vi "2D raster.vi"(11 "Scanning Parameters":T1={"x pixels"=16, "x voltage min"=-8.0, "x voltage max"=8.0, "y pixels"=16, "y voltage min"=-8.0, "y voltage max"=8.0, "x pts flyback"=16, "y pts flyback"=0, "Zoom"=1.0}) -> (1 "X and Y":waveform(dbl)[](graph)=[{"t0"=timestamp(0 s since 1904-01-01), "dt"=1.0, "Y"=array[512 elements]}, {"t0"=timestamp(0 s since 1904-01-01), "dt"=1.0, "Y"=array[512 elements]}], 2 "Y":waveform(dbl)(graph)={"t0"=timestamp(0 s since 1904-01-01), "dt"=1.0, "Y"=array[512 elements]}, 3 "X":waveform(dbl)(graph)={"t0"=timestamp(0 s since 1904-01-01), "dt"=1.0, "Y"=array[512 elements]})   [LabVIEW 2012]
panel:
  out "flyback":dbl[](graph)=[-8.0, -8.0, -8.0, -8.0, -8.0, -8.0, -10.0, -10.0, -10.0, -10.0, -10.0, -10.0, -10.0, -10.0, -10.0, -9.066666666666666]
  out "fast axis size":i32=512
  out "slow scan size":i32=512
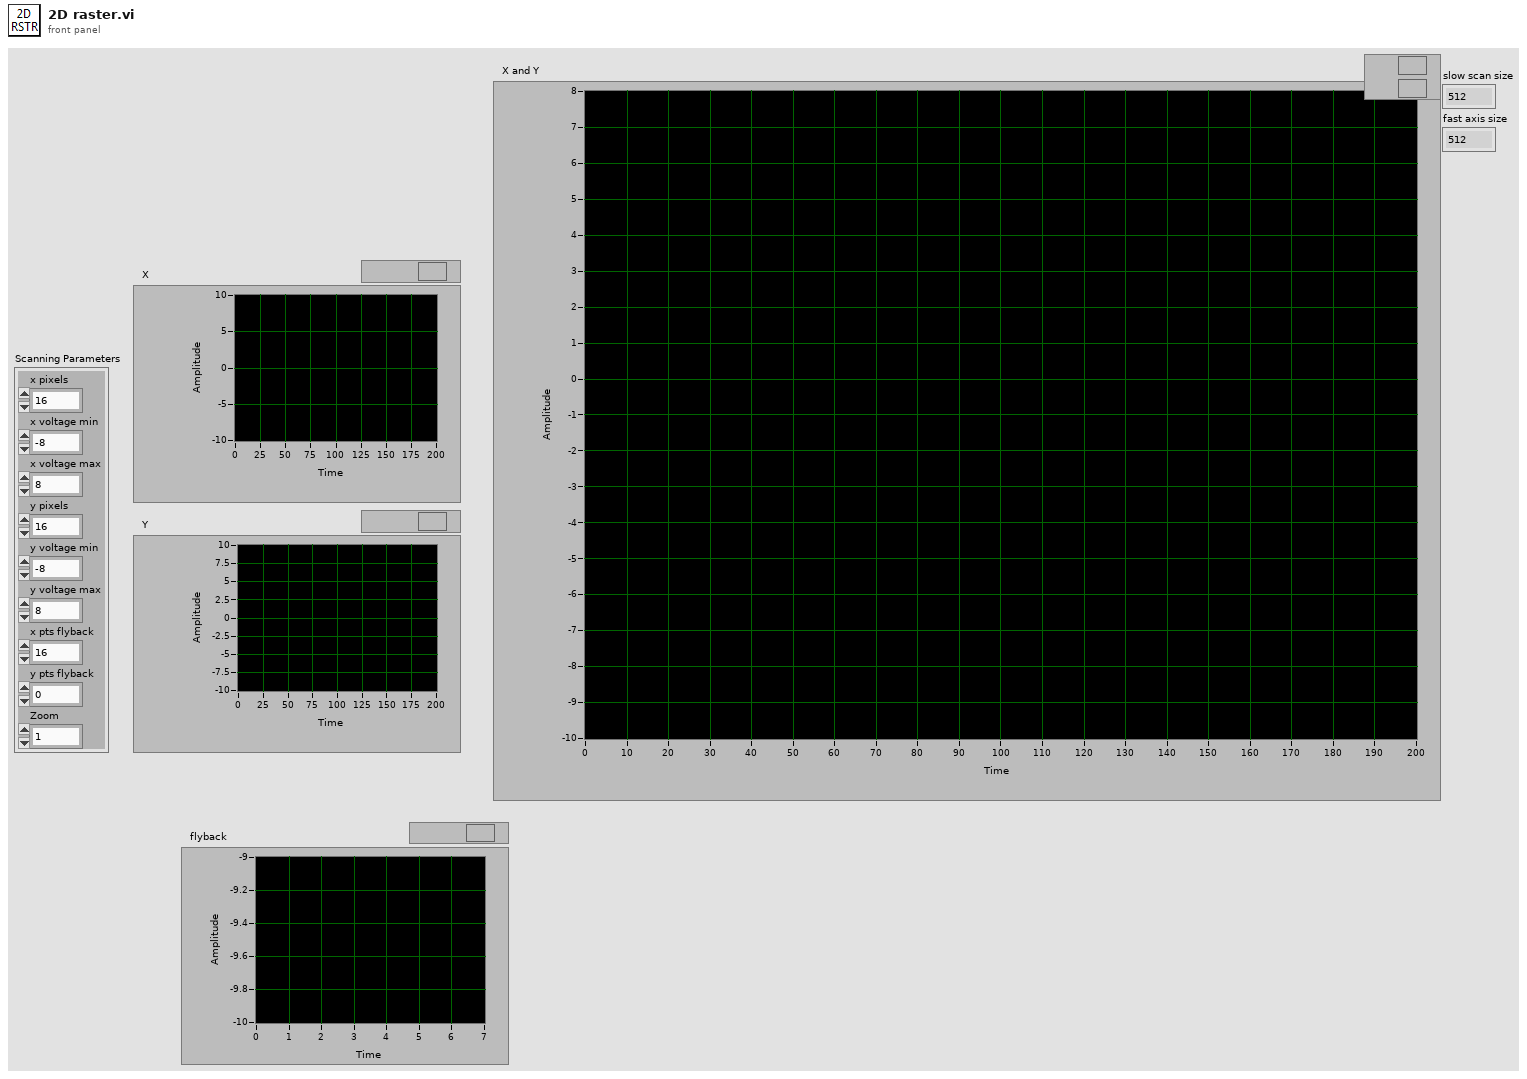
[diagram p1: front panel]
types:
  T1 = cluster{"x pixels":i32, "x voltage min":dbl, "x voltage max":dbl, "y pixels":i32, "y voltage min":dbl, "y voltage max":dbl, "x pts flyback":i32, "y pts flyback":i32, "Zoom":dbl}
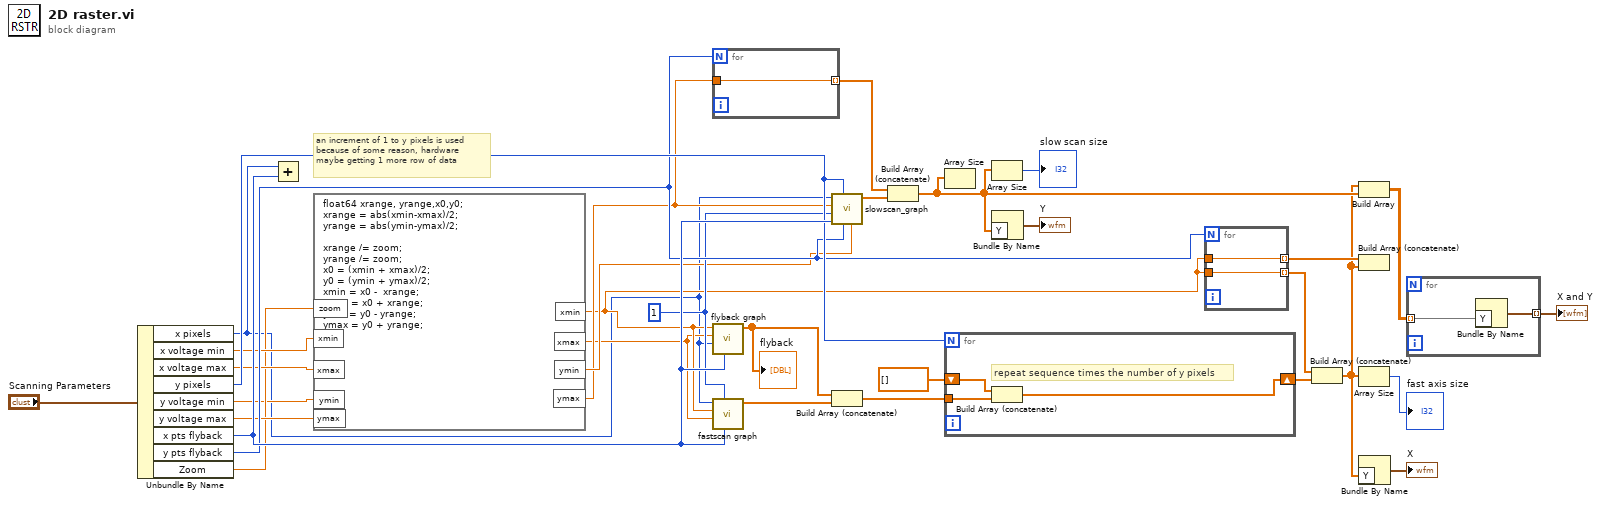
[diagram p0: block diagram]
diagram:
  w14 = 1 ("Samples to Average")
  # "an increment of 1 to y pixels is used\nbecause of some reason, hardware maybe getting 1 more row of data"
  n1 = Unbundle By Name("Scanning Parameters") -> ("x pixels"=w4:i32, "x voltage min"=w13:dbl, "x voltage max"=w12:dbl, "y pixels"=w26:i32, "y voltage min"=w9:dbl, "y voltage max"=w11:dbl, "x pts flyback"=w27:i32, "y pts flyback"=w25:i32, "Zoom"=w10:dbl)
  n2 = Add(x=w4, y=w27) -> ()  [unwired: 1 out]
  n3 = formula code="float64 xrange, yrange,x0,y0;\nxrange = abs(xmin-xmax)/2;\nyrange = abs(ymin-ymax)/2;\n\nxrange /= zoom;\nyrange /= zoom;\nx0 = (xmin + xmax)/2;\ny0 = (ymin + ymax)/2;\nxmin = x0 -  xrange;\nxmax = x0 + xrange;\nymin = y0 - yrange;\nymax = y0 + yrange;"("xmin"=w13, "xmax"=w12, "ymin"=w9, "ymax"=w11, "zoom"=w10) -> ("xmin"=w6:dbl, "xmax"=w5:dbl, "ymin"=w8:dbl, "ymax"=w7:dbl)
  n4 = for {
    N: w25 -> [_]
    tunnel: w7 -> [w33]
    tunnel: [w33] -> w24 mode=indexing
  }
  n5 = call "flyback graph.vi"("x pts flyback"=w27, "x pixels"=w4, "x max"=w5, "x min"=w6) -> ("Array"=w3:dbl[])  [unwired: 7 in]
  "flyback" <- w3
  n6 = call "fastscan graph.vi"("x pts flyback"=w27, "Samples to Average"=w14, "x max"=w5, "x min"=w6, "x pixels"=w4) -> ("Array"=w2:dbl[])  [unwired: 6 in]
  n7 = call "slowscan_graph.vi"("y min"=w8, "y pts flyback"=w25, "y pixels"=w26, "x pts flyback"=w27, "Samples to Average"=w14, "y max"=w7, "x pixels"=w4) -> ("Array out"=w23:dbl[])  [unwired: 4 in]
  n8 = Build Array (concatenate)(w3, w2) -> (w28:dbl[])
  n9 = Build Array (concatenate)(w24, w23) -> (w19:dbl[])
  n10 = Array Size(array=w19) -> ()  [unwired: 1 out]
  n11 = for {
    N: w26 -> [_]
    tunnel: w28 -> [w34]
    shift-right: [w36] -> w29
    shift-left: dbl[] [] -> [w35]
    # "repeat sequence times the number of y pixels"
    n12 = Build Array (concatenate)(w35, w34) -> (w36:dbl[])
  }
  n13 = Array Size(array=w19) -> (size(s)=→"slow scan size":i32)
  n14 = Bundle By Name("Y"=w19) -> (→"Y":waveform(dbl))  [unwired: 1 in]
  n15 = for {
    N: w25 -> [_]
    tunnel: w6 -> [w38]
    tunnel: [w38] -> w31 mode=indexing
    tunnel: [w37] -> w1 mode=indexing
    tunnel: w6 -> [w37]
  }
  n16 = Build Array (concatenate)(w1, w29) -> (w15:dbl[])
  n17 = Build Array(w15, w19) -> (w16:dbl[][])
  n18 = Build Array (concatenate)(w31, w15) -> ()  [unwired: 1 out]
  n19 = Array Size(array=w15) -> (size(s)=→"fast axis size":i32)
  n20 = Bundle By Name("Y"=w15) -> (→"X":waveform(dbl))  [unwired: 1 in]
  n21 = for {
    tunnel: w16 -> [w40] mode=indexing
    tunnel: [w39] -> w17 mode=indexing
    n22 = Bundle By Name("Y"=w40) -> (w39:waveform(dbl))  [unwired: 1 in]
  }
  "X and Y" <- w17
